vi "Create Border.vi"(7 "Infinite Point":bool, 11 "Image In":bool[][](array[boolean])) -> (3 "Image Out":bool[][](array[boolean]))   [LabVIEW 2021]
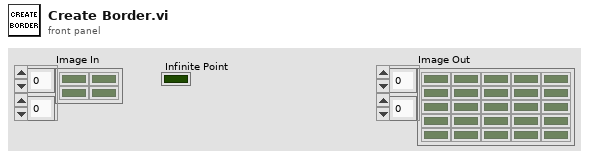
[diagram p1: front panel]
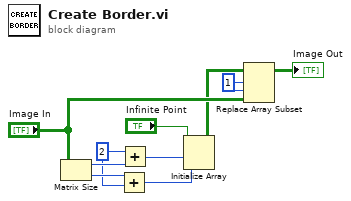
[diagram p0: block diagram]
diagram:
  w2 = 1 ("index (row)")
  w8 = 2 ("x")
  n1 = Matrix Size(0:"Image In") -> (1:w10:i32, 2:w9:i32)
  n2 = Add(x=w9, y=w8) -> (x+y=w7:i32)
  n3 = Add(x=w8, y=w10) -> (x+y=w6:i32)
  n4 = Initialize Array("Infinite Point", w6, w7) -> (w3:bool[][])
  n5 = Replace Array Subset(array=w3, new element="Image In", index (row)=w2, index (col)=w2) -> (→"Image Out":bool[][])
